vi "str to floatarray.vi"(2 "String":string) -> (6 "float array":sgl[](array[numeric]))   [LabVIEW 2014, in "OPCUA XML.lvlib"]
uses:
  OPCUA XML.lvlib
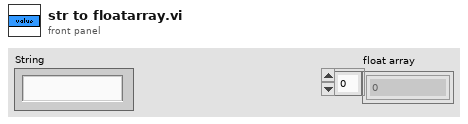
[diagram p1: front panel]
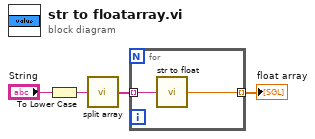
[diagram p0: block diagram]
diagram:
  n1 = To Lower Case(string="String") -> (all lower case string=w3:string)
  n2 = call "split array.vi"("string"=w3) -> ("split arr"=w2:string[])  [unwired: 8 in]
  n3 = for {
    tunnel: w2 -> [w6] mode=indexing
    tunnel: [w5] -> w1 mode=indexing
    n4 = call "str to float.vi"("String"=w6) -> ("float"=w5:sgl)  [unwired: 6 in]
  }
  "float array" <- w1
